vi "Sound Input to File.vi"() -> ()   [LabVIEW 2017]
doc: "本VI将利用麦克风输入的数据创建一个声音文件。写入文件的同时将在图形中显示声音数据。"
uses:
  <vilib>/sound2/lvsound2.llb/Sampling Mode.ctl
  <vilib>/sound2/lvsound2.llb/Sound Data Format.ctl
  <vilib>/sound2/lvsound2.llb/Sound File Write Open.vi
  <vilib>/sound2/lvsound2.llb/Sound Input Read (DBL).vi
  <vilib>/sound2/lvsound2.llb/Sound File Write (DBL).vi
panel:
  out "生成的声音文件":path
  out "波形图":waveform(dbl)[](graph)
  in  "停止":bool
  in  "设备ID":u32
  # "概述：演示使用声音函数创建一个利用麦克风输入作为数据的声音文件。\n要求：麦克风\n操作步骤：\n1. 指定设备ID的值。\n2. 运行VI。图形将显示写入至声音文件的数据。\n3.单击停止 停止VI运行。\n4.完成后删除生成的声音文件。"
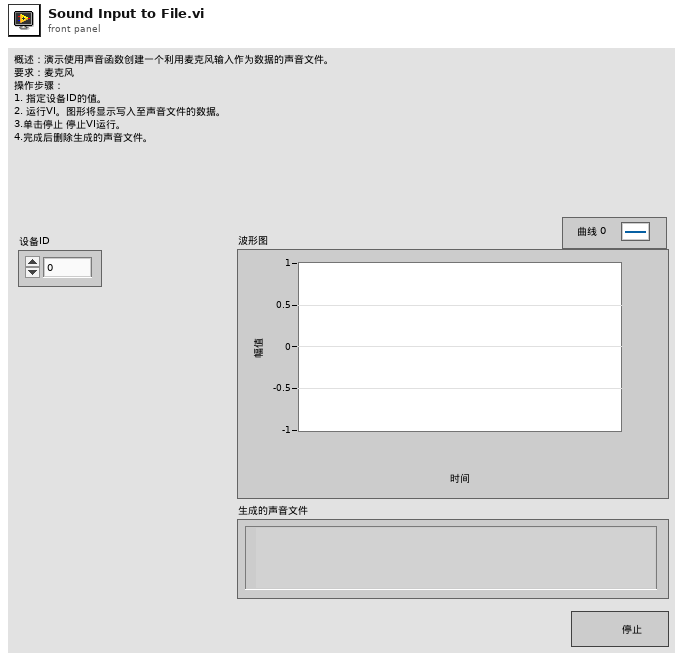
[diagram p1: front panel]
types:
  T1 = typedef "Sound Data Format.ctl" = cluster{"sample rate (S/s)":dbl, "number of channels":i32, "bits per sample":i32}
  T2 = typedef "Sampling Mode.ctl" = i32
  T3 = typedef "Sound File Refnum.ctl" = refnum<file>
  T4 = typedef "Sound Input Task ID.ctl" = u32
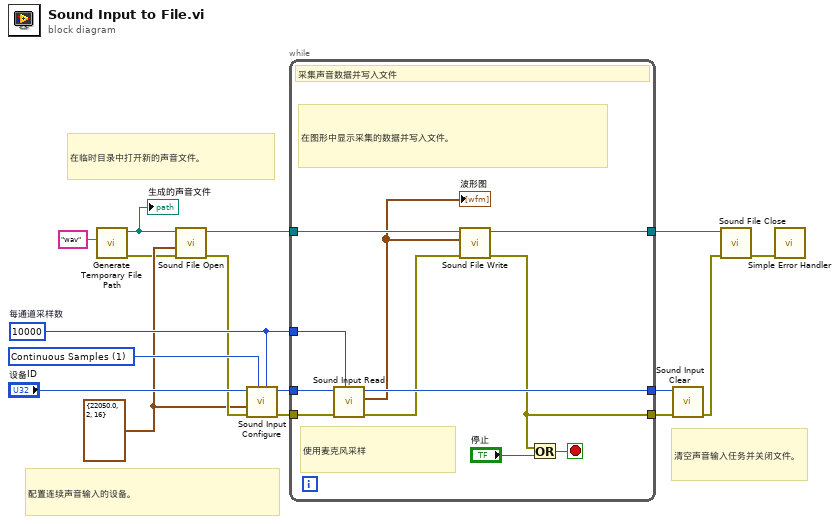
[diagram p0: block diagram]
diagram:
  w4 = T1 {"sample rate (S/s)"=22050.0, "number of channels"=2, "bits per sample"=16} ("Sound Format")
  w11 = 10000  # 每通道采样数
  w10 = T2 1 items=["Finite Samples", "Continuous Samples"] ("sample mode")
  # "配置连续声音输入的设备。"
  # "清空声音输入任务并关闭文件。"
  # "在临时目录中打开新的声音文件。"
  n1 = call <vilib>:"Generate Temporary File Path.vi"("Temporary File Extension (tmp)"="wav") -> ("error out"=w3:errorcluster, "Unique Temporary File Path"=w1:path)  [unwired: 9 in]
  "生成的声音文件" <- w1
  n2 = call-poly <vilib>:"Sound File Open.vi"("error in (no error)"=w3, "sound format"=w4, "path"=w1) -> ("error out"=w6:errorcluster, "sound file refnum"=w9:T3)  [unwired: 7 in]
  n3 = call <vilib>:"Sound Input Configure.vi"("number of samples/ch"=w11, "sample mode"=w10, "error in (no error)"=w6, "sound format"=w4, "device ID"="设备ID") -> ("error out"=w16:errorcluster, "task ID"=w14:T4)  [unwired: 5 in]
  n4 = while {
    tunnel: w11 -> [w24]
    tunnel: w9 -> [w21]
    tunnel: [w20] -> w8
    tunnel: w14 -> [w26]
    tunnel: [w25] -> w13
    tunnel: w16 -> [w27]
    tunnel: [w17] -> w12
    stop <- w22 stop-if-true
    # "使用麦克风采样"
    # "在图形中显示采集的数据并写入文件。"
    # "采集声音数据并写入文件"
    n5 = call-poly <vilib>:"Sound Input Read.vi"("number of samples/ch"=w24, "error in (no error)"=w27, "task ID"=w26) -> ("error out"=w19:errorcluster, "data"=w18:waveform(dbl)[], "task ID out"=w25:T4)  [unwired: 6 in]
    "波形图" <- w18
    n6 = call-poly <vilib>:"Sound File Write.vi"("error in (no error)"=w19, "data"=w18, "sound file refnum"=w21) -> ("error out"=w17:errorcluster, "sound file refnum out"=w20:T3)  [unwired: 7 in]
    n7 = Or(x=w17, y="停止") -> (x .or. y?=w22:bool)
  }
  n8 = call <vilib>:"Sound Input Clear.vi"("error in (no error)"=w12, "task ID"=w13) -> ("error out"=w7:errorcluster)  [unwired: 9 in]
  n9 = call <vilib>:"Sound File Close.vi"("error in (no error)"=w7, "sound file refnum"=w8) -> ("error out"=w5:errorcluster)  [unwired: 9 in]
  n10 = call <vilib>:"Simple Error Handler.vi"("error in (no error)"=w5) -> ()  [unwired: 4 in, 5 out]
